vi "FGV_PSP - VRM Remote.vi"(4 "error in":errorcluster, 6 "Function":enum16{"write", "read"}(ring), 7 "VRM Remote":bool) -> (0 "error out":errorcluster, 3 "VRM Remote":bool)   [LabVIEW 2016]
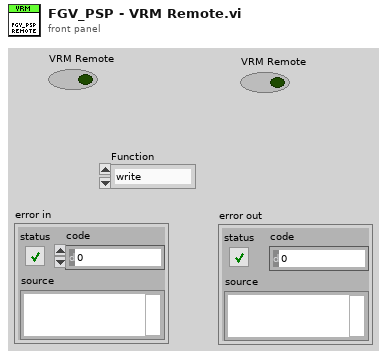
[diagram p1: front panel]
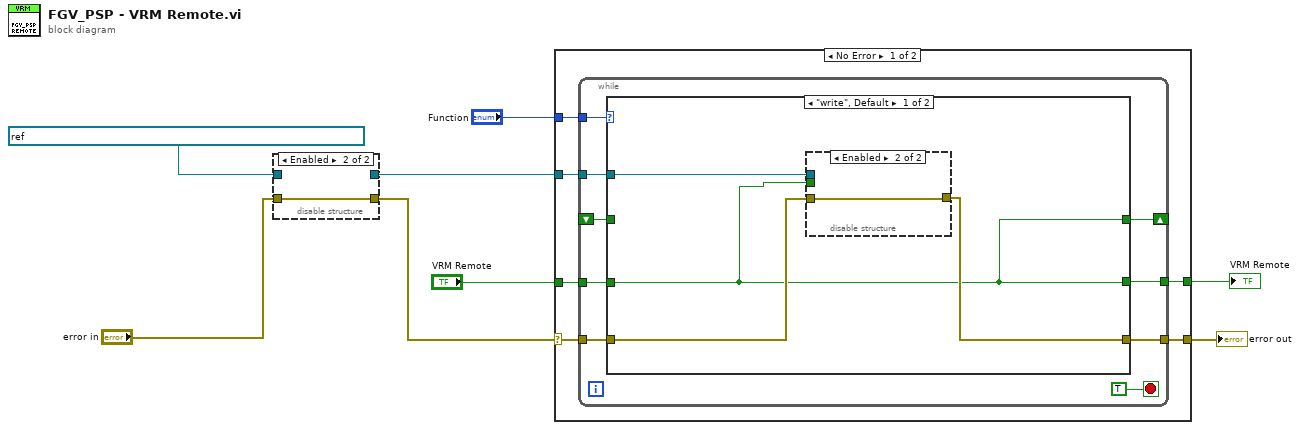
[diagram p0: block diagram]
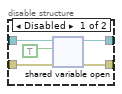
[diagram p2: hidden frame]
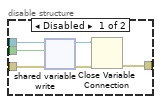
[diagram p3: hidden frame]
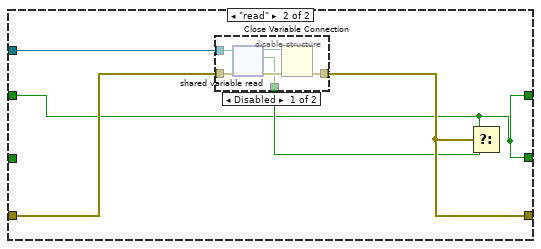
[diagram p4: hidden frame]
diagram:
  n1 = disable-structure shown="Enabled" {
    disable-tunnel: [w13 _] -> w6
    disable-tunnel: [w12 w14] -> w5
    disable-tunnel: "error in" -> [w11 w14]
    disable-tunnel: refnum<k21> "ni.var.psp://localhost/VRM/VRM_Remote" ("shared variable refnum in") -> [w9 _]
    frame Disabled {
      n2 = shared-variable-open(w9, w11, TRUE) -> (w13:refnum<k21>, w12:errorcluster)  [unwired: 1 in]
    }
    frame Enabled {
    }
  }
  n3 = case shown="No Error" w5 {
    selector: w5 -> [w20 w53]
    tunnel: [w19 w53] -> w8
    tunnel: [w18 w52] -> w1
    tunnel: "Function" -> [w17 _]
    tunnel: w6 -> [w16 _]
    tunnel: "VRM Remote" -> [w15 w52]
    frame No Error {
      n4 = while {
        shift-right: [w24] -> _
        shift-left: _ -> [w23]
        tunnel: w20 -> [w28]
        tunnel: [w27] -> w19
        tunnel: [w26] -> w18
        tunnel: w17 -> [w25]
        tunnel: w16 -> [w22]
        tunnel: w15 -> [w21]
        stop <- TRUE stop-if-true
        n5 = case shown="\"write\", Default" w25 {
          tunnel: w28 -> [w32 w44]
          tunnel: [w33 w43] -> w27
          tunnel: [w30 w41] -> w26
          tunnel: [w30 w41] -> w24
          tunnel: w23 -> [_ w41]
          tunnel: w22 -> [w31 w45]
          tunnel: w21 -> [w30 _]
          frame "write", Default {
            n6 = disable-structure shown="Enabled" {
              disable-tunnel: [w39 w40] -> w33
              disable-tunnel: w32 -> [w38 w40]
              disable-tunnel: w31 -> [w37 _]
              disable-tunnel: w30 -> [w34 _]
              frame Disabled {
                n7 = shared-variable-write(w37, w38, w34) -> (w35:refnum<k21>, w36:errorcluster)
                n8 = Close Variable Connection(8:w36, 11:w35) -> (0:w39:errorcluster)
              }
              frame Enabled {
              }
            }
          }
          frame "read" {
            n9 = disable-structure shown="Disabled" {
              disable-tunnel: w45 -> [w51 _]
              disable-tunnel: w44 -> [w50 _]
              disable-tunnel: [w49 _] -> w43
              disable-tunnel: [w46 _] -> w42
              frame Disabled {
                n10 = shared-variable-read(w51, w50) -> (w48:refnum<k21>, w47:errorcluster, w46:bool)  [unwired: 1 out]
                n11 = Close Variable Connection(8:w47, 11:w48) -> (0:w49:errorcluster)
              }
              frame Enabled {
              }
            }
            n12 = Select(t=w41, s=w43, f=w42) -> ()  [unwired: 1 out]
          }
        }
      }
    }
    frame Error {
    }
  }
  "error out" <- w8
  "VRM Remote" <- w1
